vi "3D Cartesian Coordinate Rotation (Direction) (Scalar).vi"(6 "rotation matrix type":u16(ring) items=["Direction Angles", "Direction Cosines"], 8 "Rotation Matrix":dbl[][](array[numeric]), 9 "z":dbl, 10 "y":dbl, 11 "x":dbl) -> (0 "error":i32, 1 "z out":dbl, 2 "y out":dbl, 3 "x out":dbl)   [LabVIEW 2010, in "NI_AALPro.lvlib"]
doc: "Rotates a three-dimensional Cartesian coordinate in the counterclockwise direction using the direction cosines method. Wire data to the <B>X</B> input to determine the polymorphic instance to use or manually select the instance."
uses:
  NI_AALPro.lvlib
  lvanlys.dll
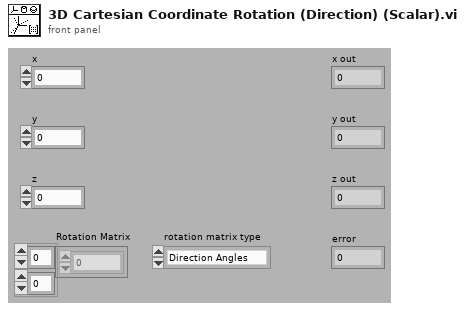
[diagram p1: front panel]
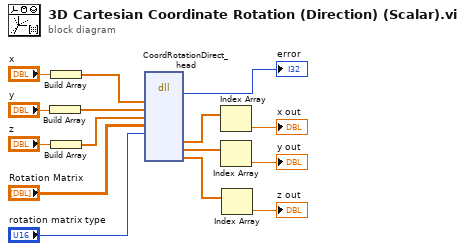
[diagram p0: block diagram]
diagram:
  n1 = Build Array("y") -> (w8:dbl[])
  n2 = Build Array("x") -> (w9:dbl[])
  n3 = Build Array("z") -> (w7:dbl[])
  n4 = dll-call lib="C:/Program Files/National Instruments/LabVIEW 2010/resource/lvanlys.*" fn="CoordRotationDirect_head"("X"=w9, "Y"=w8, "Z"=w7, "RotateMatrix"="Rotation Matrix", "param"="rotation matrix type") -> (→"error":i32, "Xout"=w4:dbl[], "Yout"=w5:dbl[], "Zout"=w6:dbl[])  [unwired: 11 in, 2 out]
  n5 = Index Array(array=w4) -> (element=→"x out":dbl)  [unwired: 1 in]
  n6 = Index Array(array=w5) -> (element=→"y out":dbl)  [unwired: 1 in]
  n7 = Index Array(array=w6) -> (element=→"z out":dbl)  [unwired: 1 in]
